vi "Format IPF GUI.vi"(10 "IPF sub folders":path[](array[path]), 11 "Inspection Program Data[]":T1[](array[typedef])) -> (3 "Item names":string[][](array[string]))   [LabVIEW 2013, in "Manipulate IPF.lvlib"]
uses:
  Manipulate IPF.lvlib
  3013/code/Modules/GUI/GUI_5/subPanels/program/type_def/Inspection program data.ctl
  3013/code/Modules/Configuration/type_def/Scan Params.ctl
  3013/code/Modules/Configuration/type_def/Profile Resolution.ctl
  3013/code/Modules/Preprocess Data/type_def/direction.ctl
  3013/code/Modules/Inspection/Data/Panel_class/type_def/Control file rel path.ctl
  3013/code/Modules/GUI/GUI_5/subPanels/edit/type_def/Description.ctl
  <userlib>/_OpenG.lib/file/file.llb/Strip Path Extension - String__ogtk.vi
  <userlib>/_OpenG.lib/string/string.llb/Convert EOLs (String)__ogtk.vi
  3013/code/Modules/Inspection/Data/Panel_class/Panel.lvclass
  3013/code/Modules/Configuration/Config.lvlib
  3013/code/Modules/Preprocess Data/PreProcess.lvlib
  3013/code/Modules/GUI/GUI_5/subPanels/program/program.lvlib
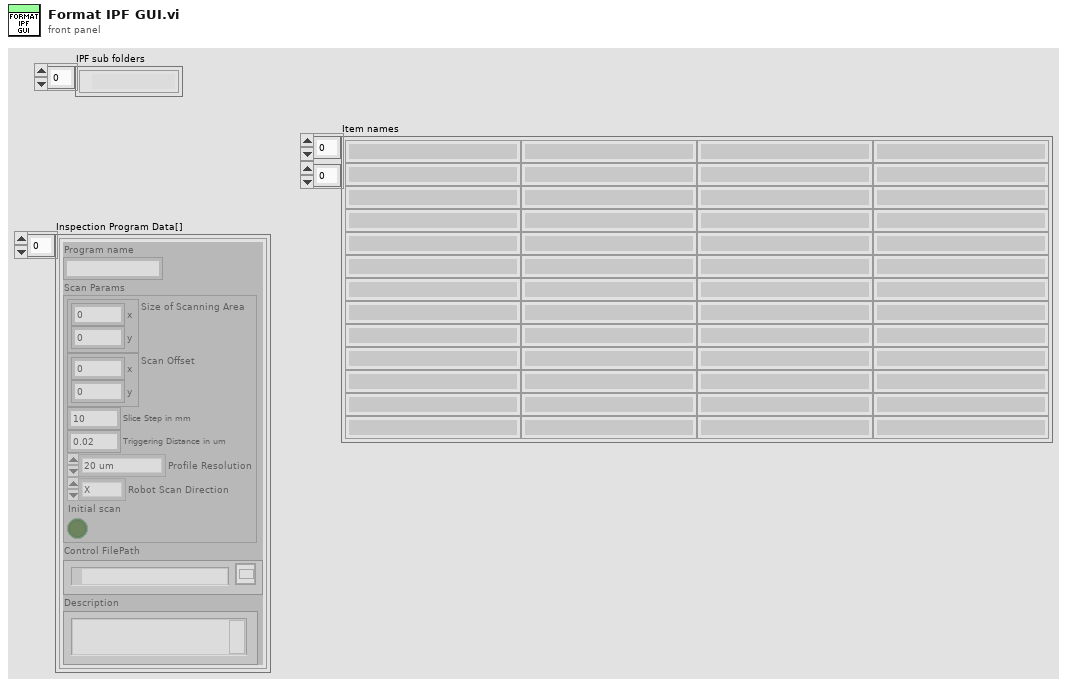
[diagram p1: front panel]
types:
  T1 = typedef "GUI.lvlib/subPanel.lvlib/program.lvlib/Inspection program data.ctl" = cluster{"Program name":string, "Scan Params":T2, "Control FilePath":T5, "Description":T6}
  T2 = typedef "Config.lvlib/Scan Params.ctl" = cluster{"Size of Scanning Area":cluster{"x":dbl, "y":dbl}, "Scan Offset":cluster{"x":dbl, "y":dbl}, "Slice Step in mm":dbl, "Triggering Distance in mm":dbl, "Triggering Distance in um":dbl, "Profile Resolution":T3, "Version":string, "Robot Scan Direction":T4, "Initial scan":bool}
  T3 = typedef "Config.lvlib/Profile Resolution.ctl" = enum8{"20 um", "40 um"}
  T4 = typedef "PreProcess.lvlib/direction.ctl" = enum8{"X", "Y"}
  T5 = typedef "Inspection.lvlib/Panel.lvclass/Control file rel path.ctl" = path
  T6 = typedef "Description.ctl" = string
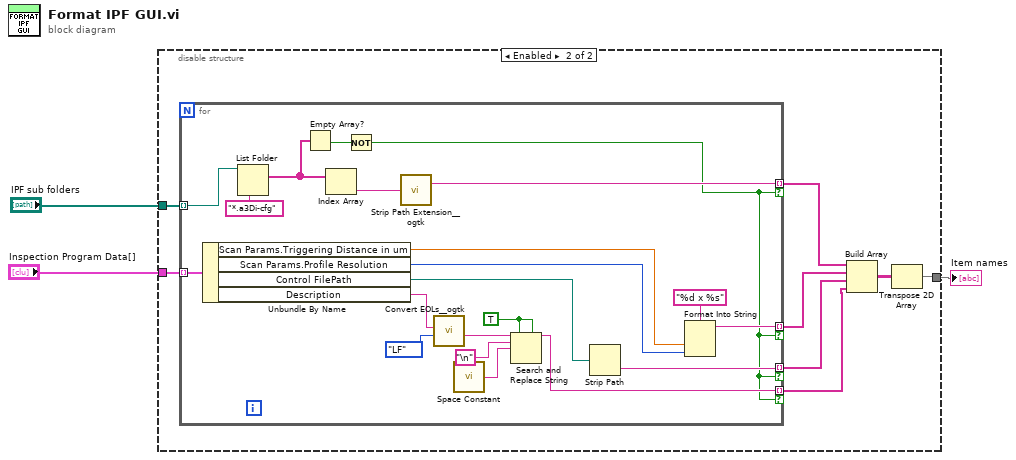
[diagram p0: block diagram]
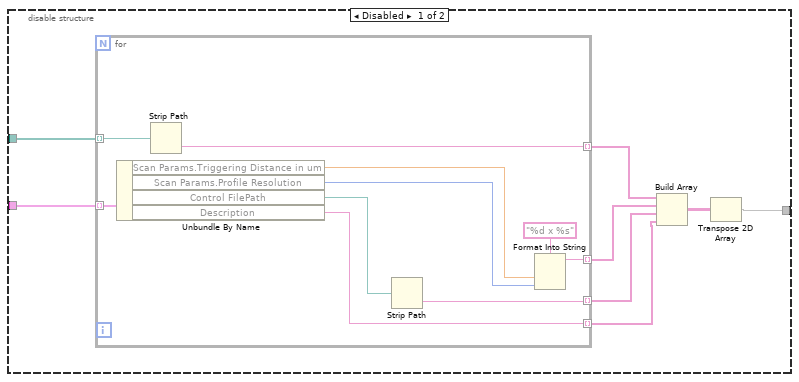
[diagram p2: hidden frame]
diagram:
  n1 = disable-structure shown="Enabled" {
    disable-tunnel: [w7 w25] -> w3
    disable-tunnel: "Inspection Program Data[]" -> [w6 w24]
    disable-tunnel: "IPF sub folders" -> [w5 w23]
    frame Disabled {
      n2 = for {
        tunnel: w6 -> [w21] mode=indexing
        tunnel: [w19] -> w8 mode=indexing
        tunnel: [w17] -> w10 mode=indexing
        tunnel: [w16] -> w11 mode=indexing
        tunnel: w5 -> [w13] mode=indexing
        tunnel: [w12] -> w4 mode=indexing
        n3 = Unbundle By Name(w21) -> ("Scan Params.Triggering Distance in um"=w15:dbl, "Scan Params.Profile Resolution"=w14:T3, "Control FilePath"=w18:T5, "Description"=w16:T6)
        n4 = Strip Path(path=w13) -> (name=w12:string)  [unwired: 1 out]
        n5 = Strip Path(path=w18) -> (name=w17:string)  [unwired: 1 out]
        n6 = Format Into String(format string="%d x %s", w15, w14) -> (resulting string=w19:string)  [unwired: 2 in, 1 out]
      }
      n7 = Build Array(w4, w8, w10, w11) -> (w9:T6[][])
      n8 = Transpose 2D Array(2D array=w9) -> (transposed array=w7:T6[][])
    }
    frame Enabled {
      n9 = for {
        tunnel: w24 -> [w50] mode=indexing
        tunnel: [w48] -> w26 mode=indexing if=w30
        tunnel: [w46] -> w28 mode=indexing if=w30
        tunnel: [w33] -> w29 mode=indexing if=w30
        tunnel: w23 -> [w43] mode=indexing
        tunnel: [w40] -> w22 mode=indexing if=w30
        w38 = TRUE ("replace all? (F)")
        n10 = Unbundle By Name(w50) -> ("Scan Params.Triggering Distance in um"=w45:dbl, "Scan Params.Profile Resolution"=w44:T3, "Control FilePath"=w47:T5, "Description"=w34:T6)
        n11 = List Folder(path=w43, pattern="*.a3Di-cfg") -> (filenames=w32:string[])  [unwired: 2 in, 3 out]
        n12 = Empty Array?(array=w32) -> (empty?=w31:bool)
        n13 = Index Array(array=w32) -> (element=w41:string)  [unwired: 1 in]
        n14 = Not(x=w31) -> (.not. x?=w30:bool)
        n15 = call-poly <userlib>:"Strip Path Extension__ogtk.vi"("path"=w41) -> ("root"=w40:string)  [unwired: 1 out]
        n16 = call-poly <userlib>:"Convert EOLs__ogtk.vi"("Convert to:"=enum16{"CR", "LF", "CRLF"}."LF", "String in"=w34) -> ("String out"=w35:string)  [unwired: 9 in]
        n17 = call <vilib>:"Space Constant.vi"() -> ("String"=w39:string)
        n18 = Search and Replace String(replace all?=w38, multiline?=w38, input string=w35, search string="\n", replace string=w39) -> (result string=w33:string)  [unwired: 3 in, 3 out]
        n19 = Strip Path(path=w47) -> (name=w46:string)  [unwired: 1 out]
        n20 = Format Into String(format string="%d x %s", w45, w44) -> (resulting string=w48:string)  [unwired: 2 in, 1 out]
      }
      n21 = Build Array(w22, w26, w28, w29) -> (w27:string[][])
      n22 = Transpose 2D Array(2D array=w27) -> (transposed array=w25:string[][])
    }
  }
  "Item names" <- w3
